vi "AlternatingLEDs.vi"() -> ()   [LabVIEW 2014]
doc: "This program alternates a high value on port 0 lines 0 and 1 to be used with a simple LED circuit to alternate LEDs until the stop button is pressed.\n\nBryan Ghahremani -SID: 1135515\nKenneth Heide -SID: 1269429"
panel:
  in  "stop":bool
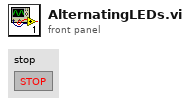
[diagram p1: front panel]
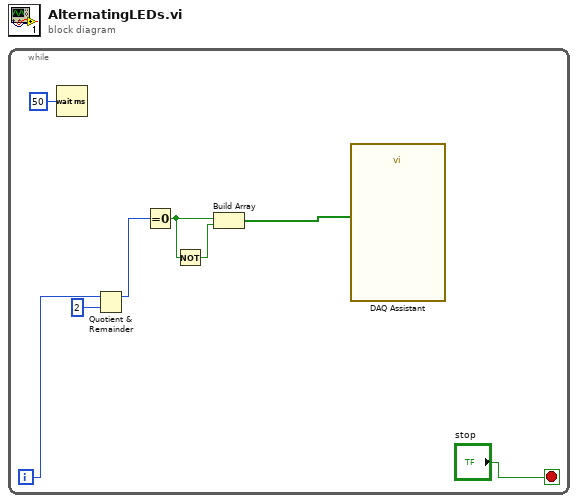
[diagram p0: block diagram]
diagram:
  n1 = while {
    i -> [w6]
    stop <- "stop" stop-if-true
    n2 = Wait (ms)(milliseconds to wait=u32 50) -> ()  [unwired: 1 out]
    n3 = Quotient & Remainder(x=w6, y=2) -> (x-y*floor(x/y)=w4:i32)  [unwired: 1 out]
    n4 = Equal To 0?(x=w4) -> (x = 0?=w3:bool)
    n5 = Not(x=w3) -> (.not. x?=w2:bool)
    n6 = Build Array(w3, w2) -> (w7:bool[])
    n7 = call "DAQ Assistant"("data"=w7) -> ()  [unwired: 17 in, 2 out]
  }
